vi "KE6514.ProcCases.vi"(0 "i ref in":refnum<vi>, 1 "selector":string, 2 "Data":T1, 3 "call cluster":T2={"Object"="", "Selector"="", "CallType"=enum."synchronous", "Async Object"="", "Async Selector"="", "Data Descriptor"="", "Data"=[], "Error #"=0, "Expire"=0}, 5 "error in (no error)":errorcluster) -> (14 "i ref out":refnum<vi>, 17 "answer cluster":T2={"Object"="", "Selector"="", "CallType"=enum."synchronous", "Async Object"="", "Async Selector"="", "Data Descriptor"="", "Data"=[], "Error #"=0, "Expire"=0}, 19 "error out":errorcluster)   [LabVIEW 2014, in "KE6514.lvlib"]
doc: "This method is called by a process from within the default case in the event loop. The methods of a class that are linked to events will be called from THIS method. Add your code here."
uses:
  KE6514.lvlib
  CS_Core/CSSystem/CoreDefs/CoreDefs.call_type.ctl
  CS_Core/BaseProcess/BaseProcess.descriptor string definition.ctl
  CS_Core/CSSystem/CoreDefs/CoreDefs.rawDataType.ctl
  CS_Core/CSSystem/CoreDefs/CoreDefs.error_type.ctl
  CS_Core/CSSystem/CoreLib/CoreLib.string 2 byte array.vi
  CS_Core/CSSystem/CoreLib/CoreLib.byte array 2 double.vi
  CS_Core/BaseProcess/BaseProcess.lvlib
  CS_Core/CSApplicationBaseClasses/DeviceBase/DeviceBase.lvlib
  CS_Core/CSSystem/CoreLib/CoreLib.lvlib
  CS_Core/CSSystem/CSSystemLib/CSSystemLib.lvlib
  CSlibraries-extern/DimLVEvent/LVDimInterface/LVDimInterface.lvlib
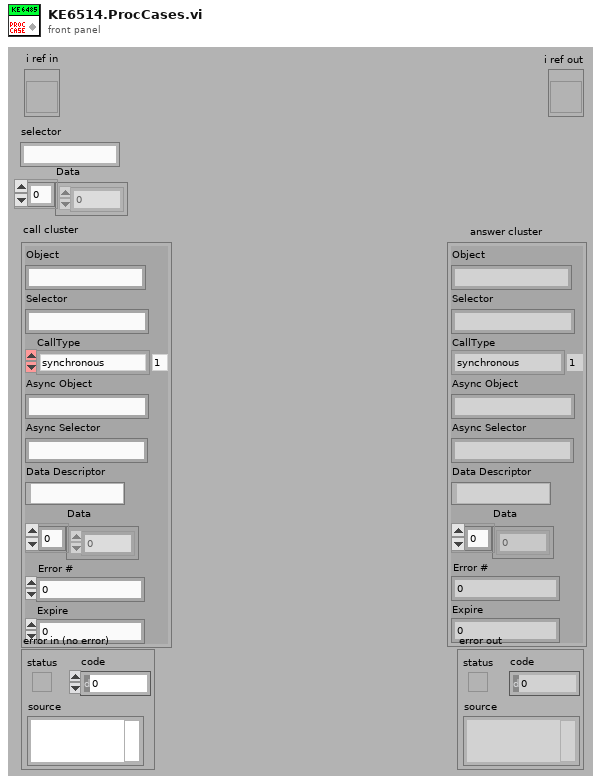
[diagram p1: front panel]
types:
  T1 = typedef "CoreDefs.rawDataType.ctl" = i8[]
  T2 = typedef "CoreDefs.call_type.ctl" = cluster{"Object":string, "Selector":string, "CallType":enum16{"simple", "synchronous", "asynchronous"}, "Async Object":string, "Async Selector":string, "Data Descriptor":T3, "Data":T1, "Error #":i32, "Expire":u32}
  T3 = typedef "BaseProcess.lvlib/BaseProcess.descriptor string definition.ctl" = string
  T4 = typedef "CoreDefs.error_type.ctl" = enum16{"no error", "can't load process", "can't unload process", "process does not exist", "can't install process", "can't remove process", "unknown function", "time out", "can't execute function", "duplicate queue name", "super not found", "caller queue invalid", "can't ping process", "unknown error", "VISA Error", "VISA timeout", "GPIB timeout", "GPIB error", "communication error", "data type mismatch", "can't read data from OPC server", "can't write data to OPC server", "OET error", "function not implemented", "process already exists", "invalid Shared Variable name", "error writing Shared Variable", "error reading Shared Variable", "invalid client name", "corrupt database", "unknown class", "call not authorized", "parameter out of range", "OET timeout: can't get data to modify", "invalid queue name", "requested operation incompatible with current state", "event undefined", "event disabled", "state undefined", "caller is not a friend", "EventBuilder: bad eventID", "EventBuilder: no DAQ devices", "a thread must not stop itself", "UNUSED ELEMENT4", "DiscArchiver: eventData incomplete", "DiscArchiver: eventData does not belong to run", "DiscArchiver: can't open file", "DiscArchiver: can't write to file", "DiscArchiver: available disc space low", "can't acquire semaphore", "error reading data from database", "notifier object is not existing", "can't register process", "can't unregister process", "illegal event type", "object disabled", "object already exists", "can't change state", "Instrument not found", "no connection to remote node", "invalid reference", "N/A", "UNUSED ELEMENT 1", "element not found", "illegal TCP/IP connection detected", "object does not exist", "invalid access ID", "unknown CS system", "invalid privilige", "unsupported data type", "unsupported server type", "IO server already exists", "Shared Variable already exists"}
  T5 = typedef "KE6514.lvlib/KE6514.i attribute.ctl" = cluster{"VISA resource name":refnum<visa-resource-name>, "ValueID":i32, "MeasurementRunning?":bool, "actSequencer":string, "actScanner":string, "actPPG":string, "MeasuredID":i32}
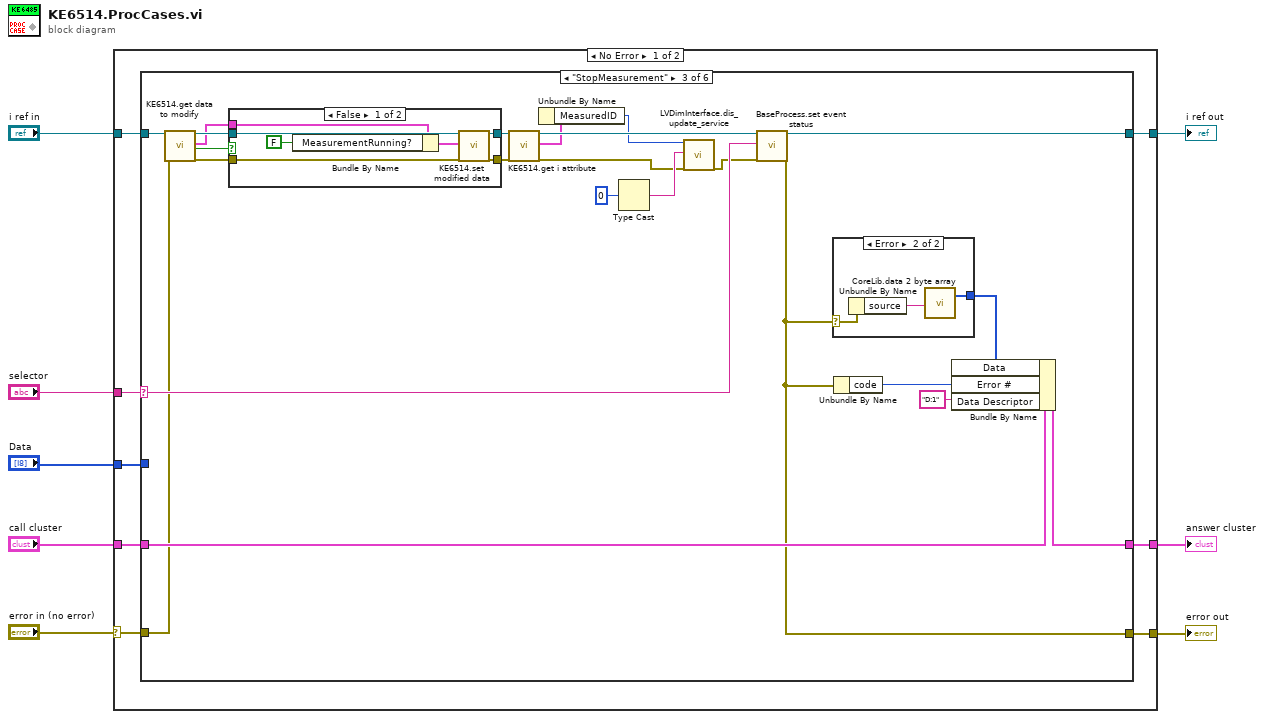
[diagram p0: block diagram]
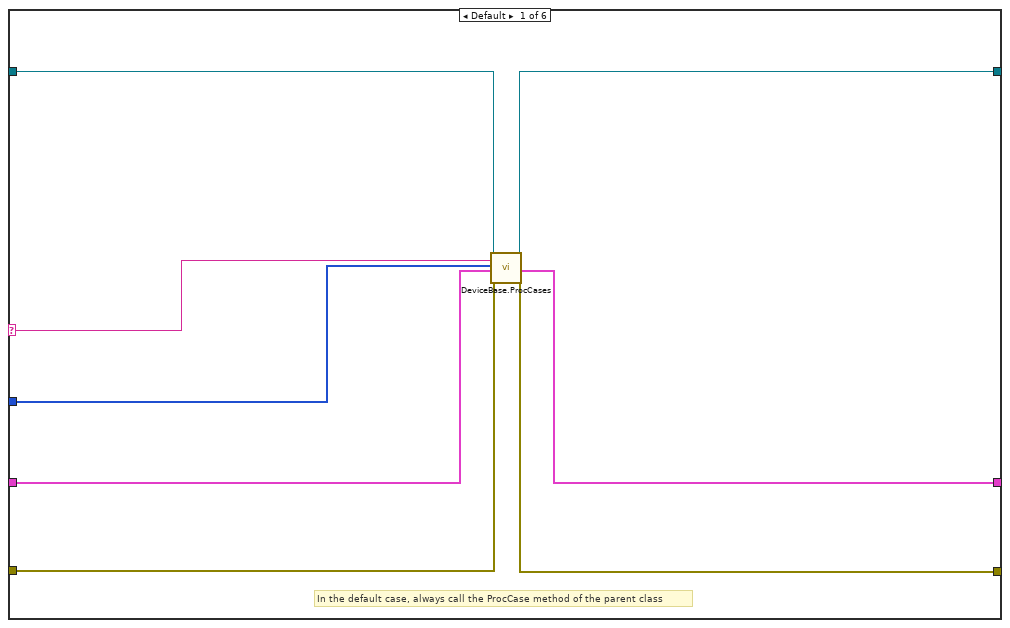
[diagram p2: hidden frame]
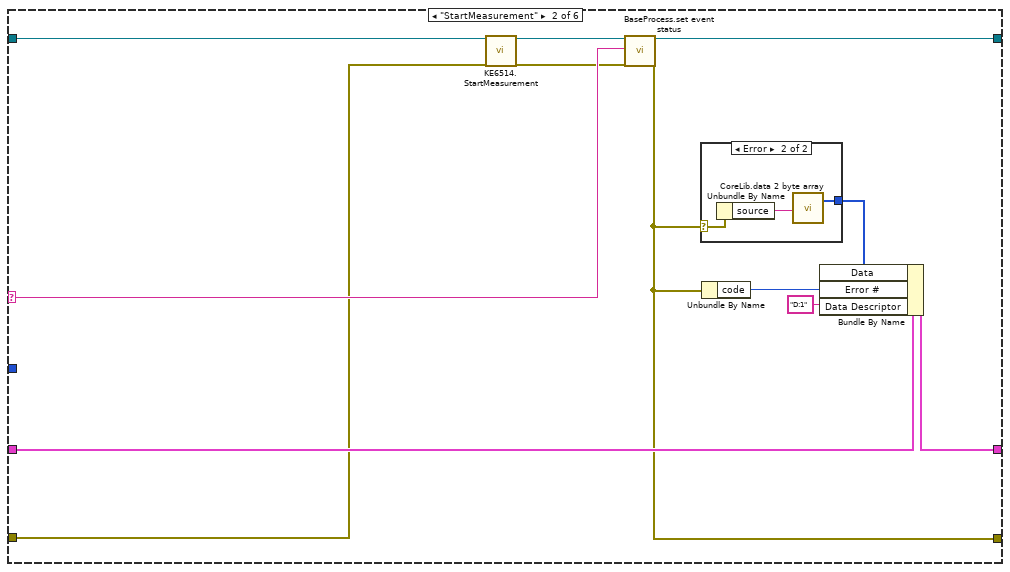
[diagram p3: hidden frame]
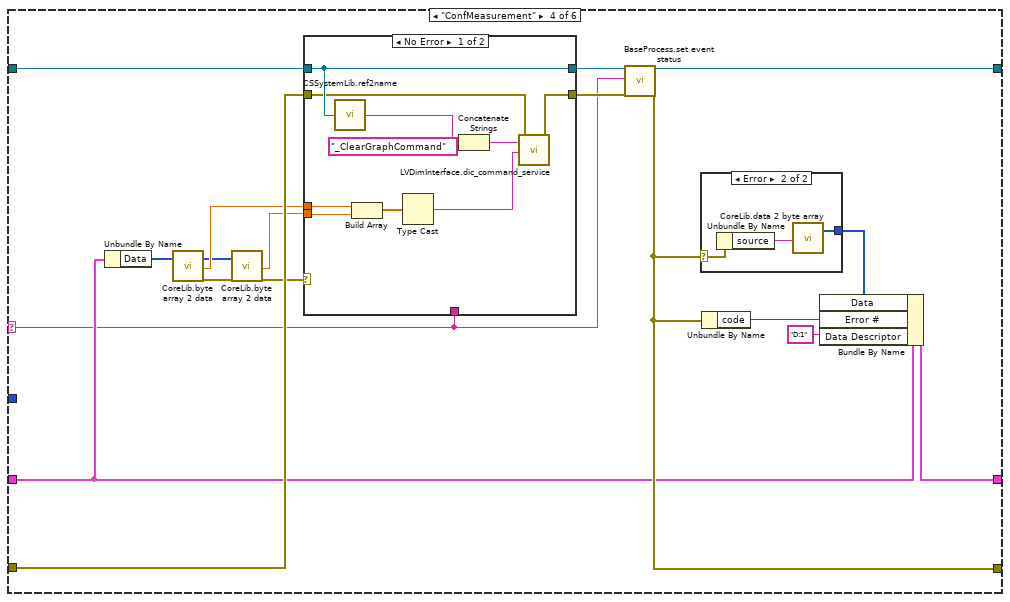
[diagram p7: hidden frame]
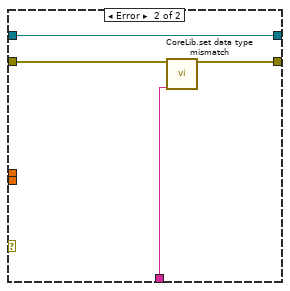
[diagram p8: hidden frame]
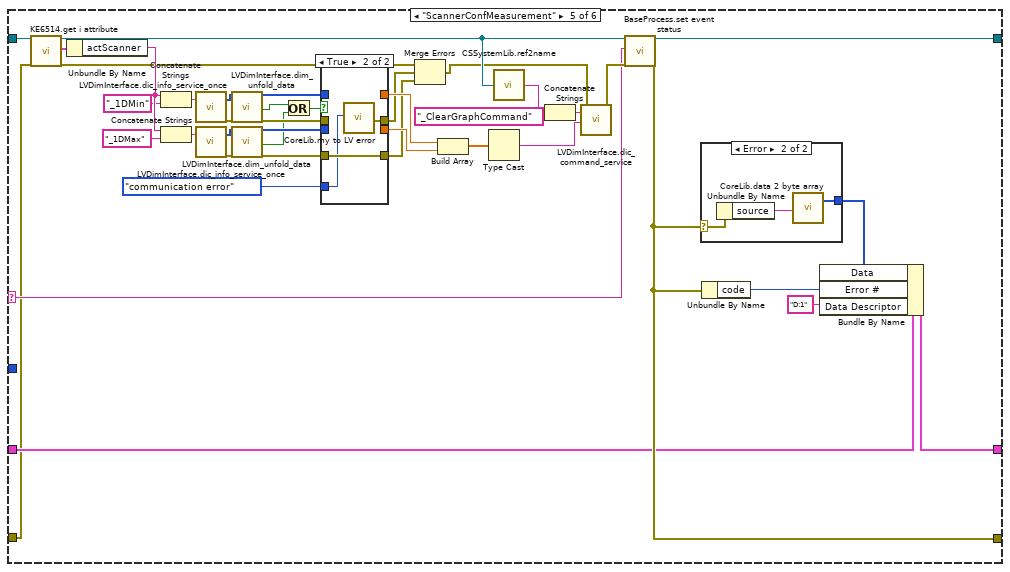
[diagram p10: hidden frame]
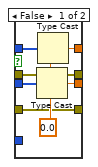
[diagram p11: hidden frame]
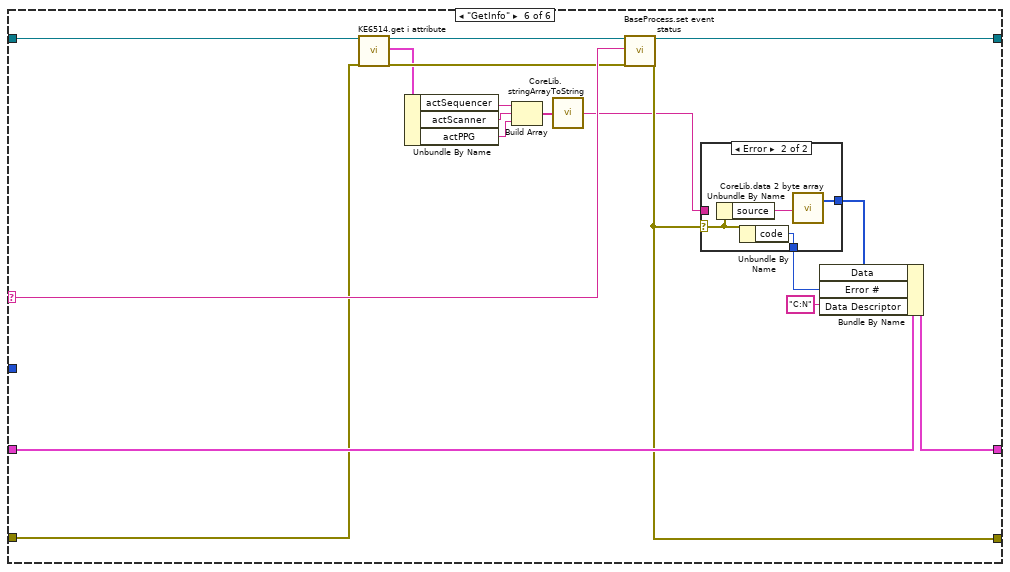
[diagram p13: hidden frame]
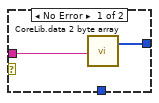
[diagram p14: hidden frame]
diagram:
  n1 = case shown="No Error" "error in (no error)" {
    selector: "error in (no error)" -> [w9 w188]
    tunnel: "selector" -> [w16 _]
    tunnel: [w15 w189] -> w7
    tunnel: "Data" -> [w14 _]
    tunnel: "call cluster" -> [w13 w189]
    tunnel: "i ref in" -> [w12 w190]
    tunnel: [w11 w190] -> w3
    tunnel: [w10 w188] -> w2
    frame No Error {
      n2 = case shown="\"StopMeasurement\"" w16 {
        selector: w16 -> [w19 w31 w57 w75 w142 w177]
        tunnel: w14 -> [w17 _ _ _ _ _]
        tunnel: w12 -> [w18 w25 w54 w83 w136 w173]
        tunnel: [w24 w30 w56 w88 w146 w176] -> w11
        tunnel: w13 -> [w20 w35 w61 w82 w143 w181]
        tunnel: [w21 w34 w60 w91 w149 w180] -> w15
        tunnel: w9 -> [w23 w28 w48 w86 w134 w174]
        tunnel: [w22 w32 w58 w89 w147 w178] -> w10
        frame Default {
          # "In the default case, always call the ProcCase method of the parent class"
          n3 = call "DeviceBase.ProcCases.vi"("i ref in"=w18, "selector"=w19, "Data"=w17, "call cluster"=w20, "error in (no error)"=w23) -> ("i ref out"=w24:refnum<vi>, "answer cluster"=w21:T2, "error out"=w22:errorcluster)  [unwired: 12 in]
        }
        frame "StartMeasurement" {
          n4 = call "KE6514.StartMeasurement.vi"("i ref in"=w25, "error in (no error)"=w28) -> ("i ref out"=w26:refnum<vi>, "error out"=w27:errorcluster)  [unwired: 16 in]
          n5 = call "BaseProcess.set event status.vi"("i ref in"=w26, "EventStatus"=w31, "error in (no error)"=w27) -> ("i ref out"=w30:refnum<vi>, "error out"=w32:errorcluster)  [unwired: 14 in, 1 out]
          n6 = case shown="Error" w32 {
            selector: w32 -> [_ w39]
            tunnel: [_ w38] -> w33
            frame No Error {
            }
            frame Error {
              n7 = Unbundle By Name(w39) -> ("source"=w37:string)
              n8 = call-poly "CoreLib.data 2 byte array.vi"("string"=w37) -> ("byteArray out"=w38:T1)  [unwired: 18 in]
            }
          }
          n9 = Unbundle By Name(w32) -> ("code"=w36:i32)
          n10 = Bundle By Name(cluster=w35, "Data"=w33, "Error #"=w36, "Data Descriptor"="D:1") -> (w34:T2)
        }
        frame "StopMeasurement" {
          n11 = call "KE6514.get data to modify.vi"("i ref in"=w54, "error in (no error)"=w48) -> ("i ref out"=w52:refnum<vi>, "i attribute"=w50:T5, "timed out"=w53:bool, "error out"=w51:errorcluster)  [unwired: 14 in]
          n12 = case shown="False" w53 {
            tunnel: [w69 w70] -> w47
            tunnel: [w68 w71] -> w45
            tunnel: w52 -> [w67 w71]
            tunnel: w51 -> [w66 w70]
            tunnel: w50 -> [w65 _]
            frame False {
              n13 = Bundle By Name(cluster=w65, "MeasurementRunning?"=FALSE) -> (w64:T5)
              n14 = call "KE6514.set modified data.vi"("i ref in"=w67, "i attribute"=w64, "error in (no error)"=w66) -> ("i ref out"=w68:refnum<vi>, "error out"=w69:errorcluster)  [unwired: 15 in]
            }
            frame True {
            }
          }
          n15 = call "KE6514.get i attribute.vi"("i ref in"=w45, "error in (no error)"=w47) -> ("i ref out"=w44:refnum<vi>, "i attribute"=w41:T5, "error out"=w46:errorcluster)  [unwired: 15 in]
          n16 = Unbundle By Name(w41) -> ("MeasuredID"=w40:i32)
          n17 = Type Cast(x=i16 0) -> (*(type *) &x=w49:string)  [unwired: 1 in]
          n18 = call "LVDimInterface.dis_update_service.vi"("my_serviceID"=w40, "data"=w49, "error in (no error)"=w46) -> ("error out"=w43:errorcluster)  [unwired: 14 in, 2 out]
          n19 = call "BaseProcess.set event status.vi"("i ref in"=w44, "EventStatus"=w57, "error in (no error)"=w43) -> ("i ref out"=w56:refnum<vi>, "error out"=w58:errorcluster)  [unwired: 14 in, 1 out]
          n20 = case shown="Error" w58 {
            selector: w58 -> [_ w74]
            tunnel: [_ w73] -> w59
            frame No Error {
            }
            frame Error {
              n21 = Unbundle By Name(w74) -> ("source"=w72:string)
              n22 = call-poly "CoreLib.data 2 byte array.vi"("string"=w72) -> ("byteArray out"=w73:T1)  [unwired: 18 in]
            }
          }
          n23 = Unbundle By Name(w58) -> ("code"=w62:i32)
          n24 = Bundle By Name(cluster=w61, "Data"=w59, "Error #"=w62, "Data Descriptor"="D:1") -> (w60:T2)
        }
        frame "ConfMeasurement" {
          n25 = Unbundle By Name(w82) -> ("Data"=w80:T1)
          n26 = call-poly "CoreLib.byte array 2 data.vi"("byteArray"=w80) -> ("byteArray out"=w77:T1, "d64"=w78:dbl, "error out"=w81:errorcluster)  [unwired: 16 in]
          n27 = call-poly "CoreLib.byte array 2 data.vi"("byteArray"=w77, "error in (no error)"=w81) -> ("d64"=w76:dbl, "error out"=w79:errorcluster)  [unwired: 15 in, 1 out]
          n28 = case shown="No Error" w79 {
            tunnel: w86 -> [w98 w106]
            tunnel: [w97 w105] -> w85
            tunnel: [w100 w104] -> w84
            tunnel: w83 -> [w100 w104]
            tunnel: w78 -> [w96 _]
            tunnel: w76 -> [w95 _]
            tunnel: w75 -> [_ w103]
            frame No Error {
              n29 = call "CSSystemLib.ref2name.vi"("obj refnum"=w100) -> ("name"=w101:string)
              n30 = Build Array(w96, w95) -> (w94:dbl[])
              n31 = Type Cast(x=w94) -> (*(type *) &x=w93:string)  [unwired: 1 in]
              n32 = Concatenate Strings(w101, "_ClearGraphCommand" ("string")) -> (w99:string)
              n33 = call "LVDimInterface.dic_command_service.vi"("commandName"=w99, "data"=w93, "error in (no error)"=w98) -> ("error out"=w97:errorcluster)  [unwired: 15 in, 1 out]
            }
            frame Error {
              n34 = call "CoreLib.set data type mismatch.vi"("error in (no error)"=w106, "error source"=w103) -> ("error out"=w105:errorcluster)  [unwired: 17 in]
            }
          }
          n35 = call "BaseProcess.set event status.vi"("i ref in"=w84, "EventStatus"=w75, "error in (no error)"=w85) -> ("i ref out"=w88:refnum<vi>, "error out"=w89:errorcluster)  [unwired: 14 in, 1 out]
          n36 = case shown="Error" w89 {
            selector: w89 -> [_ w109]
            tunnel: [_ w108] -> w90
            frame No Error {
            }
            frame Error {
              n37 = Unbundle By Name(w109) -> ("source"=w107:string)
              n38 = call-poly "CoreLib.data 2 byte array.vi"("string"=w107) -> ("byteArray out"=w108:T1)  [unwired: 18 in]
            }
          }
          n39 = Unbundle By Name(w89) -> ("code"=w92:i32)
          n40 = Bundle By Name(cluster=w82, "Data"=w90, "Error #"=w92, "Data Descriptor"="D:1") -> (w91:T2)
        }
        frame "ScannerConfMeasurement" {
          n41 = call "KE6514.get i attribute.vi"("i ref in"=w136, "error in (no error)"=w134) -> ("i ref out"=w135:refnum<vi>, "i attribute"=w133:T5, "error out"=w121:errorcluster)  [unwired: 15 in]
          n42 = Unbundle By Name(w133) -> ("actScanner"=w132:string)
          n43 = Concatenate Strings(w132, "_1DMin" ("string")) -> (w129:string)
          n44 = Concatenate Strings(w132, "_1DMax" ("string")) -> (w128:string)
          n45 = call "LVDimInterface.dic_info_service_once.vi"("serviceName"=w129) -> ("data"=w127:i8[], "error out"=w119:errorcluster)  [unwired: 15 in, 2 out]
          n46 = call "LVDimInterface.dic_info_service_once.vi"("serviceName"=w128) -> ("data"=w126:i8[], "error out"=w118:errorcluster)  [unwired: 15 in, 2 out]
          n47 = call "LVDimInterface.dim_unfold_data.vi"("rawData"=w127, "error in (no error)"=w119) -> ("data"=w125:i8[], "no link"=w112:bool, "error out"=w115:errorcluster)  [unwired: 14 in, 1 out]
          n48 = call "LVDimInterface.dim_unfold_data.vi"("rawData"=w126, "error in (no error)"=w118) -> ("data"=w124:i8[], "no link"=w111:bool, "error out"=w117:errorcluster)  [unwired: 14 in, 1 out]
          n49 = Or(x=w112, y=w111) -> (x .or. y?=w113:bool)
          n50 = case shown="True" w113 {
            tunnel: w125 -> [w157 _]
            tunnel: w124 -> [w156 _]
            tunnel: [w154 _] -> w123
            tunnel: [w153 _] -> w122
            tunnel: w117 -> [w152 w159]
            tunnel: [w152 w159] -> w116
            tunnel: w115 -> [w151 _]
            tunnel: [w151 w160] -> w114
            tunnel: CoreDefs.error_type."communication error" ("ErrorTypes") -> [_ w158]
            frame False {
              w155 = 0.0
              n51 = Type Cast(type=w155, x=w156) -> (*(type *) &x=w153:dbl)
              n52 = Type Cast(type=w155, x=w157) -> (*(type *) &x=w154:dbl)
            }
            frame True {
              n53 = call "CoreLib.my to LV error.vi"("ErrorTypes"=w158) -> ("myErrorCluster"=w160:errorcluster)  [unwired: 17 in, 1 out]
            }
          }
          n54 = Merge Errors(w121, w114, w116) -> (w120:errorcluster)
          n55 = Build Array(w123, w122) -> (w138:dbl[])
          n56 = Type Cast(x=w138) -> (*(type *) &x=w137:string)  [unwired: 1 in]
          n57 = call "CSSystemLib.ref2name.vi"("obj refnum"=w135) -> ("name"=w140:string)
          n58 = Concatenate Strings(w140, "_ClearGraphCommand" ("string")) -> (w139:string)
          n59 = call "LVDimInterface.dic_command_service.vi"("commandName"=w139, "data"=w137, "error in (no error)"=w120) -> ("error out"=w144:errorcluster)  [unwired: 15 in, 1 out]
          n60 = call "BaseProcess.set event status.vi"("i ref in"=w135, "EventStatus"=w142, "error in (no error)"=w144) -> ("i ref out"=w146:refnum<vi>, "error out"=w147:errorcluster)  [unwired: 14 in, 1 out]
          n61 = case shown="Error" w147 {
            selector: w147 -> [_ w163]
            tunnel: [_ w162] -> w148
            frame No Error {
            }
            frame Error {
              n62 = Unbundle By Name(w163) -> ("source"=w161:string)
              n63 = call-poly "CoreLib.data 2 byte array.vi"("string"=w161) -> ("byteArray out"=w162:T1)  [unwired: 18 in]
            }
          }
          n64 = Unbundle By Name(w147) -> ("code"=w150:i32)
          n65 = Bundle By Name(cluster=w143, "Data"=w148, "Error #"=w150, "Data Descriptor"="D:1") -> (w149:T2)
        }
        frame "GetInfo" {
          n66 = call "KE6514.get i attribute.vi"("i ref in"=w173, "error in (no error)"=w174) -> ("i ref out"=w171:refnum<vi>, "i attribute"=w170:T5, "error out"=w172:errorcluster)  [unwired: 15 in]
          n67 = Unbundle By Name(w170) -> ("actSequencer"=w169:string, "actScanner"=w168:string, "actPPG"=w167:string)
          n68 = Build Array(w169, w168, w167) -> (w166:string[])
          n69 = call "CoreLib.stringArrayToString.vi"("Array"=w166) -> ("String"=w165:string)
          n70 = call "BaseProcess.set event status.vi"("i ref in"=w171, "EventStatus"=w177, "error in (no error)"=w172) -> ("i ref out"=w176:refnum<vi>, "error out"=w178:errorcluster)  [unwired: 14 in, 1 out]
          n71 = case shown="Error" w178 {
            selector: w178 -> [_ w185]
            tunnel: [w183 w187] -> w179
            tunnel: w165 -> [w182 _]
            tunnel: [_ w184] -> w164
            frame No Error {
              n72 = call-poly "CoreLib.data 2 byte array.vi"("string"=w182) -> ("byteArray out"=w183:T1)  [unwired: 18 in]
            }
            frame Error {
              n73 = Unbundle By Name(w185) -> ("source"=w186:string)
              n74 = Unbundle By Name(w185) -> ("code"=w184:i32)
              n75 = call-poly "CoreLib.data 2 byte array.vi"("string"=w186) -> ("byteArray out"=w187:T1)  [unwired: 18 in]
            }
          }
          n76 = Bundle By Name(cluster=w181, "Data"=w179, "Error #"=w164, "Data Descriptor"="C:N") -> (w180:T2)
        }
      }
    }
    frame Error {
    }
  }
  "answer cluster" <- w7
  "i ref out" <- w3
  "error out" <- w2
